vi "Refnums.vi"() -> ()   [LabVIEW 2016]
panel:
  in  "Compressor":string="Lift"
  in  "Lights":string="Lift"
  in  "Limit":string="wench"
  in  "Encoder":string="joystick1"
  in  "Lift":string="Lift"
  in  "Solenoid":string="Solenoid"
  in  "Gunner":string="joystick1"
  in  "Driver":string="joystick"
  in  "Wench":string="wench"
  in  "Left 3":string="left3"
  in  "Left 2":string="left2"
  in  "Left 1":string="left1"
  in  "Right 3":string="right3"
  in  "Right 2":string="right2"
  in  "Right 1":string="right1"
  # "PWM"
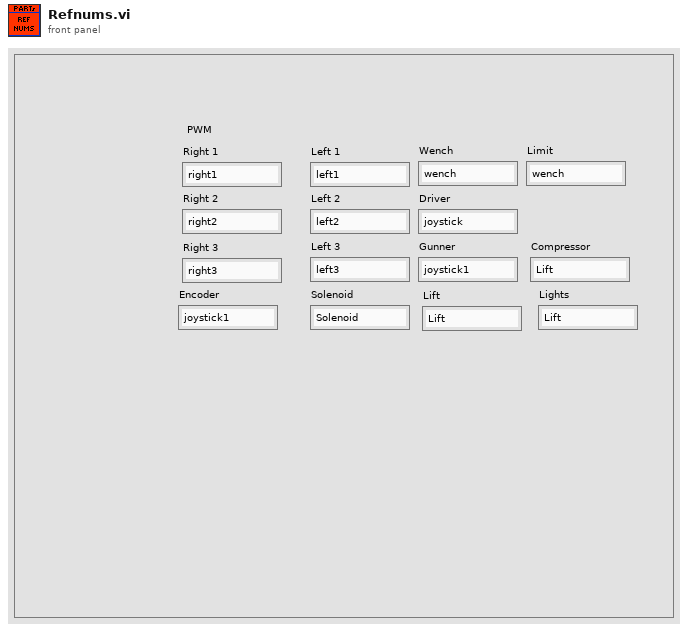
[diagram p1: front panel]
diagram:
